vi "Get Identity.vi"(8 "error in (no error)":errorcluster, 11 "User in":refnum<class "User.lvclass">) -> (0 "error out":errorcluster, 2 "Identity":string, 3 "User out":refnum<class "User.lvclass">)   [LabVIEW 2020, in "HTTP Server.lvlib" / "User.lvclass"]
uses:
  User.lvclass
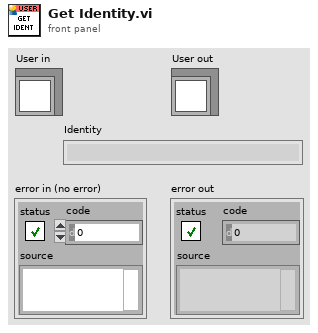
[diagram p1: front panel]
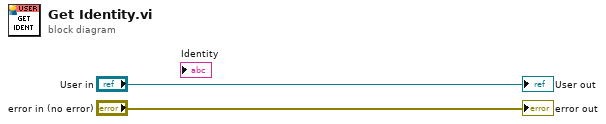
[diagram p0: block diagram]
diagram:
  "error out" <- "error in (no error)"
  "User out" <- "User in"
